vi "SupplyPowerReadout.vi"(0 "Handle In":i32, 1 "Solenoid Supply Pin":u16, 2 "LabJack Supply Pin":u16, 3 "error in":errorcluster, 4 "Relay Supply Pin":u16) -> (5 "Solenoid Supply Voltage":dbl, 6 "LabJack Supply Voltage":dbl, 7 "Relay Supply Voltage":dbl, 8 "error out":errorcluster[](array[cluster]))   [LabVIEW 2021]
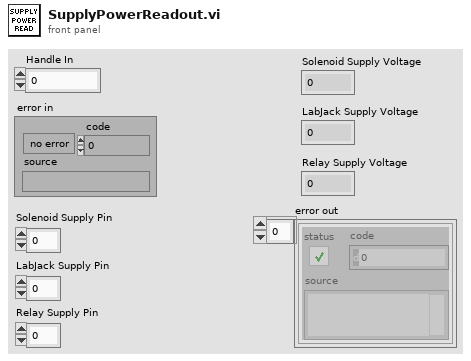
[diagram p1: front panel]
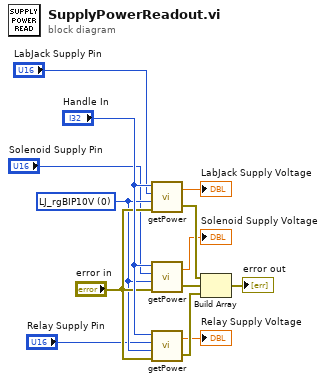
[diagram p0: block diagram]
diagram:
  w11 = u16 0 items=["LJ_rgBIP10V", "LJ_rgBIP1V", "LJ_rgBIPP1V", "LJ_rgBIPP01V"] ("AIN Range")
  n1 = call "getPower.vi"("error in"="error in", "AIN Range"=w11, "+Channel"="LabJack Supply Pin", "Handle In"="Handle In") -> ("error out"=w10:errorcluster, "Voltage Reading"=→"LabJack Supply Voltage":dbl)
  n2 = call "getPower.vi"("error in"="error in", "AIN Range"=w11, "+Channel"="Solenoid Supply Pin", "Handle In"="Handle In") -> ("error out"=w9:errorcluster, "Voltage Reading"=→"Solenoid Supply Voltage":dbl)
  n3 = call "getPower.vi"("error in"="error in", "AIN Range"=w11, "+Channel"="Relay Supply Pin", "Handle In"="Handle In") -> ("error out"=w8:errorcluster, "Voltage Reading"=→"Relay Supply Voltage":dbl)
  n4 = Build Array(w10, w9, w8) -> (→"error out":errorcluster[])
